vi "Write REM IO VARs.vi"(7 "R/W Case":T7, 8 "error in (no error)":errorcluster, 9 "Input FIFO buffer in":dbl[](array[numeric]), 10 "I/O Input Data In":T1 {"BD Refs"."Data Reference" format="%.0x"}, 11 "I/O Imput Vars in":T4[](array[typedef]) {"VS ref" format="%.0x"}) -> (0 "error out":errorcluster, 1 "Input FIFO buffer out":dbl[](array[numeric]), 2 "I/O Input Data Out":T1 {"BD Refs"."Data Reference" format="%.0x"}, 3 "I/O Imput Vars out":T4[](array[typedef]) {"VS ref" format="%.0x"})   [LabVIEW 2016, in "Scan Engine Custom Device.lvlib"]
uses:
  Scan Engine Custom Device.lvlib
  Type Defs/RW Case.ctl
  Type Defs/REM IO ECAT Slave IOV Cluster.ctl
  <vilib>/NI Veristand/Custom Device API/Custom Device Item Ref.ctl
  Type Defs/UDV Data Type.ctl
  Type Defs/Input Data.ctl
  <vilib>/NI Veristand/Custom Device API/Block Data Reference.ctl
  <vilib>/NI Veristand/Custom Device API/Data Reference.ctl
  <vilib>/NI Veristand/Custom Device API/Global Data Refs.vi
  <vilib>/NI Veristand/Custom Device API/Custom Device API.lvlib
  <vilib>/NI Veristand/Custom Device Tools/Custom Device Utility Library/Custom Device Utility Library.lvlib
  <vilib>/NI_Real-Time Target Support.lvlib
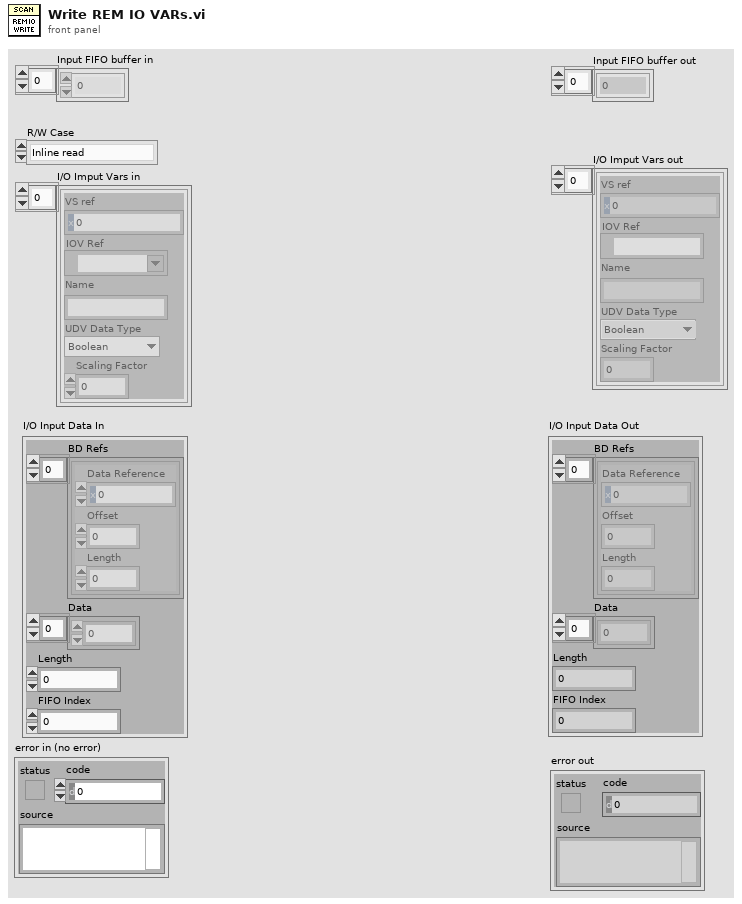
[diagram p1: front panel]
types:
  T1 = typedef "Scan Engine Custom Device.lvlib/Input Data.ctl" = cluster{"BD Refs":T2[], "Data":dbl[], "Length":i32, "FIFO Index":i32}
  T2 = typedef "Custom Device API.lvlib/Block Data Reference.ctl" = cluster{"Data Reference":T3, "Offset":u64, "Length":u64}
  T3 = typedef "Custom Device API.lvlib/Data Reference.ctl" = i32
  T4 = typedef "Scan Engine Custom Device.lvlib/REM IO ECAT Slave IOV Cluster.ctl" = cluster{"VS ref":T5, "IOV Ref":refnum<k21>, "Name":string, "UDV Data Type":T6, "Scaling Factor":dbl}
  T5 = typedef "Custom Device API.lvlib/Custom Device Item Ref.ctl" = u64
  T6 = typedef "Scan Engine Custom Device.lvlib/UDV Data Type.ctl" = enum16{"Boolean", "Fixed Point", "Int8", "Int16", "Int32", "Int64", "U32 Bit Field", "UInt8", "UInt16", "UInt32", "UInt64", "Other"}
  T7 = typedef "Scan Engine Custom Device.lvlib/RW Case.ctl" = enum16{"Inline read", "Inline write", "Async - Inline loop read", "Async - Inline loop write", "Async loop (read/write)"}
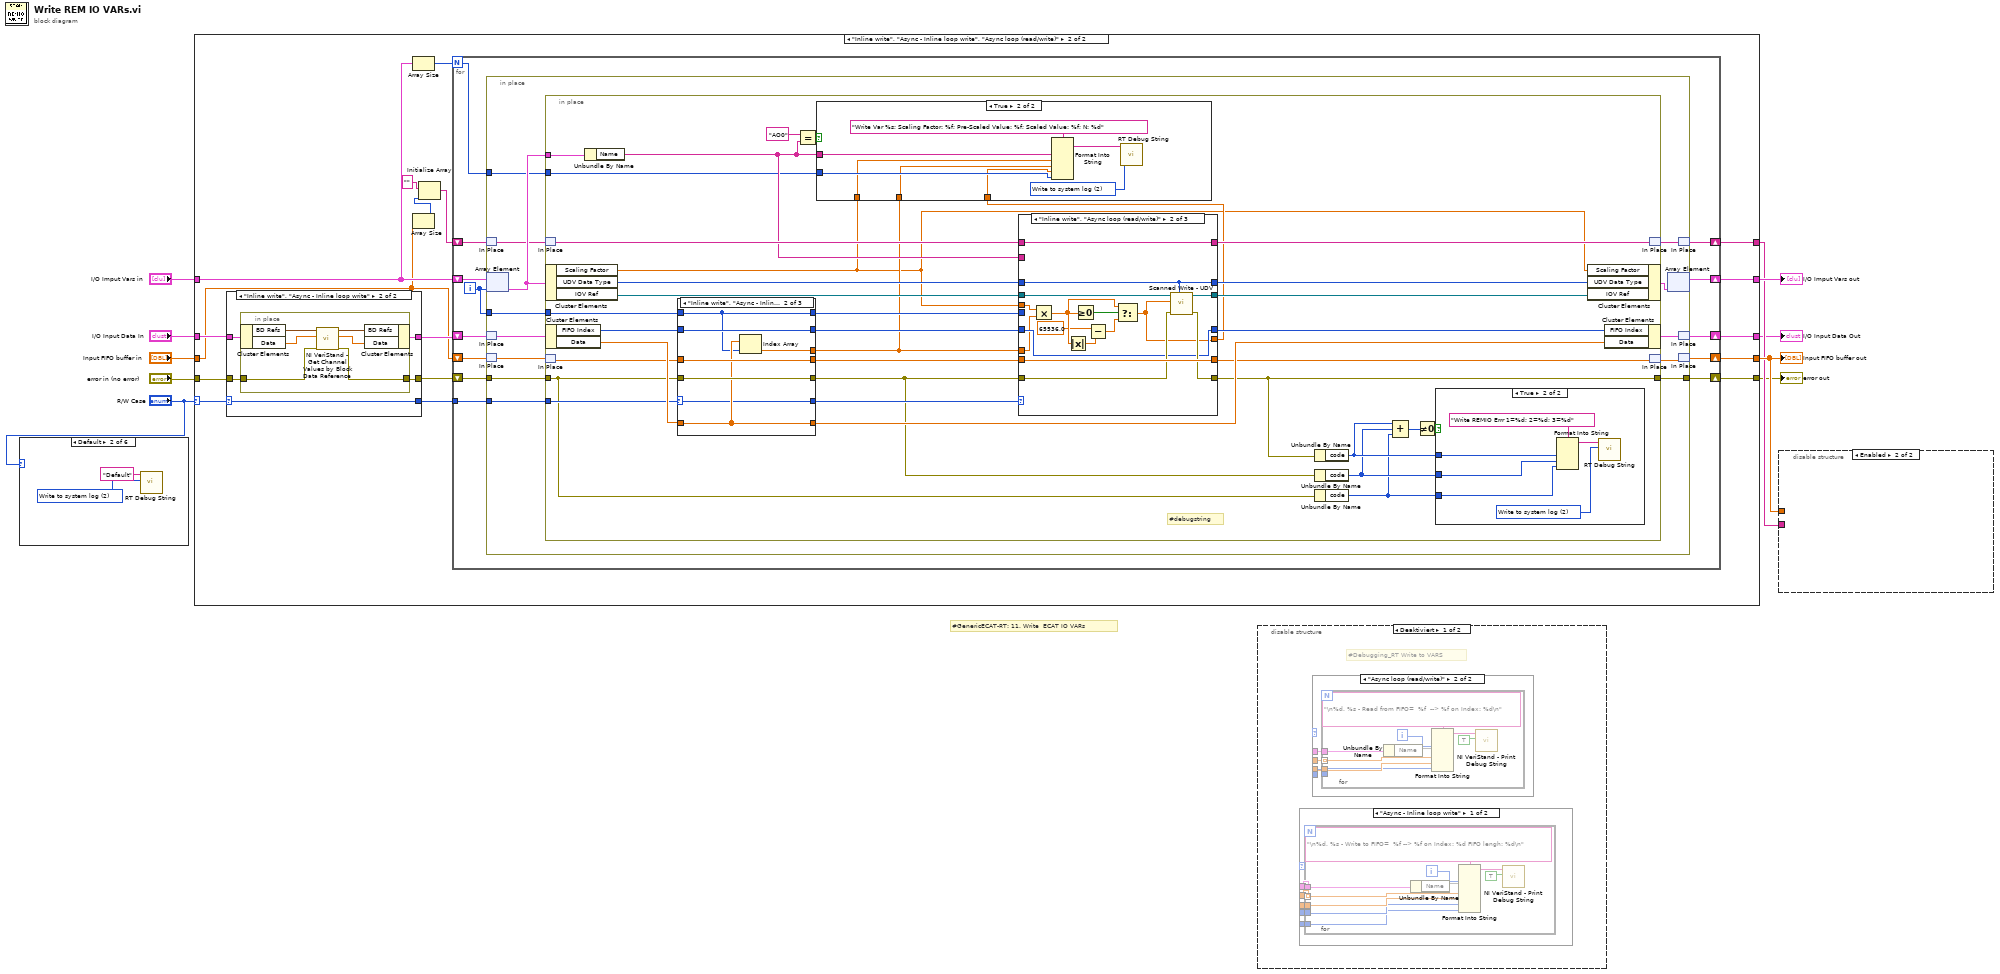
[diagram p0: block diagram]
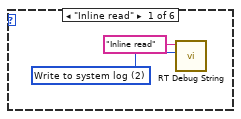
[diagram p2: hidden frame]
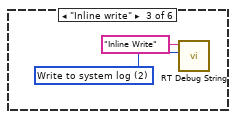
[diagram p3: hidden frame]
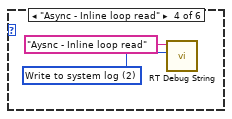
[diagram p4: hidden frame]
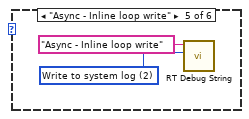
[diagram p5: hidden frame]
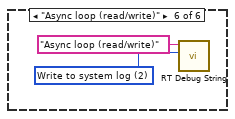
[diagram p6: hidden frame]
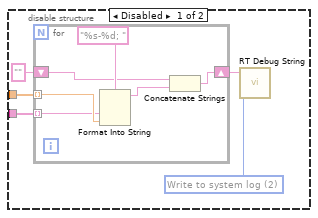
[diagram p7: hidden frame]
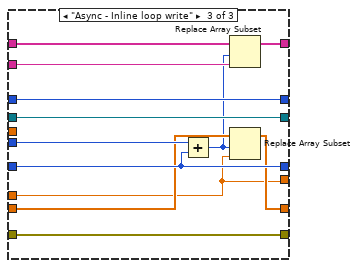
[diagram p12: hidden frame]
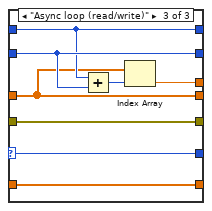
[diagram p14: hidden frame]
diagram:
  # "#GenericECAT-RT: 11. Write  ECAT IO VARs"
  n1 = case shown="Default" "R/W Case" {
    frame "Inline read" {
      w11 = u16 2 items=["Write to serial", "Write to monitor", "Write to system log"] ("Interface")
      n2 = call <vilib>:"RT Debug String.vi"("Interface"=w11, "String to write"="Inline read") -> ()  [unwired: 9 in, 1 out]
    }
    frame Default {
      w14 = u16 2 items=["Write to serial", "Write to monitor", "Write to system log"] ("Interface")
      n3 = call <vilib>:"RT Debug String.vi"("Interface"=w14, "String to write"="Default") -> ()  [unwired: 9 in, 1 out]
    }
    frame "Inline write" {
      w16 = u16 2 items=["Write to serial", "Write to monitor", "Write to system log"] ("Interface")
      n4 = call <vilib>:"RT Debug String.vi"("Interface"=w16, "String to write"="Inline Write") -> ()  [unwired: 9 in, 1 out]
    }
    frame "Async - Inline loop read" {
      w18 = u16 2 items=["Write to serial", "Write to monitor", "Write to system log"] ("Interface")
      n5 = call <vilib>:"RT Debug String.vi"("Interface"=w18, "String to write"="Aysnc - Inline loop read") -> ()  [unwired: 9 in, 1 out]
    }
    frame "Async - Inline loop write" {
      w19 = u16 2 items=["Write to serial", "Write to monitor", "Write to system log"] ("Interface")
      n6 = call <vilib>:"RT Debug String.vi"("Interface"=w19, "String to write"="Async - Inline loop write") -> ()  [unwired: 9 in, 1 out]
    }
    frame "Async loop (read/write)" {
      w21 = u16 2 items=["Write to serial", "Write to monitor", "Write to system log"] ("Interface")
      n7 = call <vilib>:"RT Debug String.vi"("Interface"=w21, "String to write"="Async loop (read/write)") -> ()  [unwired: 9 in, 1 out]
    }
  }
  n8 = case shown="\"Inline write\", \"Async - Inline loop write\", \"Async loop (read/write)\"" "R/W Case" {
    selector: "R/W Case" -> [_ w39]
    tunnel: [w24 w43] -> w6
    tunnel: "Input FIFO buffer in" -> [w24 w31]
    tunnel: [w25 w33] -> w2
    tunnel: [w26 w42] -> w7
    tunnel: "I/O Input Data In" -> [w25 w37]
    tunnel: "I/O Imput Vars in" -> [w26 w41]
    tunnel: [w23 w32] -> w4
    tunnel: "error in (no error)" -> [w23 w38]
    tunnel: [_ w28] -> w5
    frame Default {
    }
    frame "Inline write", "Async - Inline loop write", "Async loop (read/write)" {
      n9 = case shown="\"Inline write\", \"Async - Inline loop write\"" w39 {
        selector: w39 -> [w174 w177]
        tunnel: w37 -> [w175 w181]
        tunnel: w38 -> [w176 w180]
        tunnel: [w176 w179] -> w35
        tunnel: [w175 w178] -> w36
        tunnel: [w174 w177] -> w34
        frame Default {
        }
        frame "Inline write", "Async - Inline loop write" {
          n10 = in-place {
            in-place-border: w180 -> [w183]
            in-place-border: [w182] -> w179
            n11 = in-place-cluster #1(w181) -> ("BD Refs"=w187:T2[], "Data"=w185:dbl[])
            n12 = call <vilib>:"NI VeriStand - Get Channel Values by Block Data Reference.vi"("error in (no error)"=w183, "Values Array in"=w185, "Block Data Ref"=w187) -> ("error out"=w182:errorcluster, "Values Array out"=w184:dbl[], "Block Data Ref dup"=w186:T2[])  [unwired: 6 in]
            n13 = in-place-cluster #1("BD Refs"=w186, "Data"=w184) -> (w178:T1)
          }
        }
      }
      n14 = Array Size(array=w41) -> (size(s)=w40:i32)
      n15 = Array Size(array=w31) -> (size(s)=w30:i32)
      n16 = Initialize Array("", w30) -> (w27:string[])
      n17 = for {
        N: w40 -> [w44]
        shift-right: [w55] -> w42
        shift-left: w41 -> [w56]
        shift-right: [w47] -> w33
        shift-left: w36 -> [w50]
        shift-right: [w53] -> w43
        shift-left: w31 -> [w54]
        shift-right: [w51] -> w32
        shift-left: w35 -> [w52]
        tunnel: w34 -> [w49]
        shift-right: [w46] -> w28
        shift-left: w27 -> [w45]
        i -> [w48]
        n18 = in-place {
          in-place-border: w52 -> [w67]
          in-place-border: [w61] -> w51
          in-place-border: w49 -> [w66]
          in-place-border: w48 -> [w65]
          in-place-border: w44 -> [w57]
          n19 = in-place-match #2(w45) -> (w59:string[])
          n20 = in-place-array #3(w56, w48) -> (w60:T4)
          n21 = in-place-match #4(w50) -> (w69:T1)
          n22 = in-place-match #5(w54) -> (w68:dbl[])
          n23 = in-place {
            in-place-border: w67 -> [w84]
            in-place-border: w66 -> [w91]
            in-place-border: w65 -> [w102]
            in-place-border: [w82] -> w61
            in-place-border: w60 -> [w89]
            in-place-border: w57 -> [w73]
            # "#debugstring"
            n24 = in-place-match #6(w59) -> (w87:string[])
            n25 = in-place-cluster #7(w60) -> ("Scaling Factor"=w70:dbl, "UDV Data Type"=w88:T6, "IOV Ref"=w97:refnum<k21>)
            n26 = in-place-cluster #8(w69) -> ("FIFO Index"=w85:i32, "Data"=w103:dbl[])
            n27 = in-place-match #9(w68) -> (w93:dbl[])
            n28 = Unbundle By Name(w89) -> ("Name"=w76:string)
            n29 = case shown="\"Inline write\", \"Async - Inline loop write\"" w91 {
              selector: w91 -> [w155 w160 w169]
              tunnel: w102 -> [w153 w161 w170]
              tunnel: w85 -> [w158 w163 w171]
              tunnel: w93 -> [w156 w164 w168]
              tunnel: w84 -> [w154 w165 w173]
              tunnel: w103 -> [w157 w162 w172]
              tunnel: [w158 w163 w171] -> w98
              tunnel: [w157 w162 w172] -> w94
              tunnel: [w154 w165 w173] -> w83
              tunnel: [w156 w164 w168] -> w90
              tunnel: [w155 w160 w169] -> w96
              tunnel: [_ w159 w167] -> w72
              tunnel: [w153 w161 w170] -> w95
              frame Default {
              }
              frame "Inline write", "Async - Inline loop write" {
                n30 = Index Array(array=w162, index=w161) -> (element=w159:dbl)
              }
              frame "Async loop (read/write)" {
                n31 = Add(x=w170, y=w171) -> (x+y=w166:i32)
                n32 = Index Array(array=w168, index=w166) -> (element=w167:dbl)
              }
            }
            n33 = Equal?(x="AO0", y=w76) -> (x = y?=w74:bool)
            n34 = case shown="\"Inline write\", \"Async loop (read/write)\"" w96 {
              tunnel: w88 -> [w120 w137 w152]
              tunnel: w97 -> [w121 w139 w147]
              tunnel: w98 -> [w122 w128 w149]
              tunnel: w90 -> [w123 w140 w148]
              tunnel: [w123 w140 w146] -> w92
              tunnel: w95 -> [_ _ w150]
              tunnel: [w122 w128 w149] -> w99
              tunnel: [w121 w138 w147] -> w100
              tunnel: [w120 w137 w152] -> w101
              tunnel: w83 -> [w124 w136 w151]
              tunnel: [w124 w135 w151] -> w82
              tunnel: w72 -> [w118 w125 w141]
              tunnel: w87 -> [w119 w134 w145]
              tunnel: w76 -> [_ _ w143]
              tunnel: [w119 w134 w144] -> w86
              tunnel: w70 -> [_ w126 _]
              tunnel: [w118 w127 w141] -> w71
              frame Default {
              }
              frame "Inline write", "Async loop (read/write)" {
                n35 = Multiply(x=w126, y=w125) -> (x*y=w133:dbl)
                n36 = Absolute Value(x=w133) -> (abs(x)=w132:dbl)
                n37 = Greater Or Equal To 0?(x=w133) -> (x >= 0?=w129:bool)
                n38 = Subtract(x=65536.0 ("scaled data"), y=w132) -> (x-y=w131:dbl)
                n39 = Select(t=w133, s=w129, f=w131) -> (s? t:f=w127:dbl)
                n40 = call "Scanned Write - UDV.vi"("UDV Data Type"=w137, "error in (no error)"=w136, "data in"=w127, "IOV ref in"=w139) -> ("error out"=w135:errorcluster, "IOV ref out"=w138:refnum<k21>)  [unwired: 6 in]
              }
              frame "Async - Inline loop write" {
                n41 = Add(x=w150, y=w149) -> (x+y=w142:i32)
                n42 = Replace Array Subset(array=w145, new element=w143, index=w142) -> (w144:string[])
                n43 = Replace Array Subset(array=w148, new element=w141, index=w142) -> (w146:dbl[])
              }
            }
            n44 = case shown="True" w74 {
              tunnel: w72 -> [_ w104]
              tunnel: w71 -> [_ w106]
              tunnel: w76 -> [_ w111]
              tunnel: w73 -> [_ w107]
              tunnel: w70 -> [_ w105]
              frame False {
              }
              frame True {
                w110 = u16 2 items=["Write to serial", "Write to monitor", "Write to system log"] ("Interface")
                n45 = Format Into String(format string="Write Var %s; Scaling Factor: %f; Pre-Scaled Value: %f; Scaled Value: %f; N: %d", w111, w105, w104, w106, w107) -> (resulting string=w109:string)  [unwired: 2 in, 1 out]
                n46 = call <vilib>:"RT Debug String.vi"("Interface"=w110, "String to write"=w109) -> ()  [unwired: 9 in, 1 out]
              }
            }
            n47 = Unbundle By Name(w82) -> ("code"=w79:i32)
            n48 = Unbundle By Name(w83) -> ("code"=w78:i32)
            n49 = Unbundle By Name(w84) -> ("code"=w77:i32)
            n50 = Compound Arithmetic op=ADD(w79, w78, w77) -> (w81:i32)
            n51 = Not Equal To 0?(x=w81) -> (x != 0?=w80:bool)
            n52 = case shown="True" w80 {
              tunnel: w79 -> [_ w117]
              tunnel: w78 -> [_ w116]
              tunnel: w77 -> [_ w115]
              frame False {
              }
              frame True {
                w112 = u16 2 items=["Write to serial", "Write to monitor", "Write to system log"] ("Interface")
                n53 = Format Into String(format string="Write REMIO Errr 1=%d; 2=%d; 3=%d", w117, w116, w115) -> (resulting string=w113:string)  [unwired: 2 in, 1 out]
                n54 = call <vilib>:"RT Debug String.vi"("Interface"=w112, "String to write"=w113) -> ()  [unwired: 9 in, 1 out]
              }
            }
            n55 = in-place-cluster #7("Scaling Factor"=w70, "UDV Data Type"=w101, "IOV Ref"=w100) -> (w64:T4)
            n56 = in-place-cluster #8("FIFO Index"=w99, "Data"=w94) -> (w63:T1)
            n57 = in-place-match #6(w86) -> (w58:string[])
            n58 = in-place-match #9(w92) -> (w62:dbl[])
          }
          n59 = in-place-array #3(w64) -> (w55:T4[])  [unwired: 1 out]
          n60 = in-place-match #2(w58) -> (w46:string[])
          n61 = in-place-match #4(w63) -> (w47:T1)
          n62 = in-place-match #5(w62) -> (w53:dbl[])
        }
      }
    }
  }
  "Input FIFO buffer out" <- w6
  "error out" <- w4
  "I/O Imput Vars out" <- w7
  "I/O Input Data Out" <- w2
  n63 = disable-structure shown="Deaktiviert" {
    frame Disabled {
      # "#Debugging_RT Write to VARS"
      n64 = case shown="\"Async - Inline loop write\"" {
        selector: _ -> [_ _]
        tunnel: _ -> [w205 _]
        tunnel: _ -> [w204 _]
        tunnel: _ -> [w203 _]
        tunnel: _ -> [w202 _]
        tunnel: _ -> [w201 _]
        frame "Async - Inline loop write" {
          n65 = for {
            tunnel: w205 -> [w211]
            tunnel: w204 -> [w210] mode=indexing
            tunnel: w203 -> [w208]
            tunnel: w202 -> [w207]
            tunnel: w201 -> [w206]
            i -> [w213]
            n66 = Unbundle By Name(w211) -> ("Name"=w212)
            n67 = Format Into String(format string="\n%d. %s - Write to FIFO=  %f --> %f on Index: %d FIFO lengh: %d\n" ("Format-String"), w213, w212, w210, w208, w207, w206) -> (resulting string=w214:string)  [unwired: 2 in, 1 out]
            n68 = call <vilib>:"NI VeriStand - Print Debug String.vi"("Add to log file? (T)"=TRUE, "Message"=w214) -> ()  [unwired: 9 in, 1 out]
          }
        }
        frame Default {
        }
      }
      n69 = case shown="\"Async loop (read/write)\"" {
        selector: _ -> [_ _]
        tunnel: _ -> [_ w191]
        tunnel: _ -> [_ w190]
        tunnel: _ -> [_ w189]
        tunnel: _ -> [_ w188]
        frame "Async - Inline loop write", Default {
        }
        frame "Async loop (read/write)" {
          n70 = for {
            tunnel: w191 -> [w195]
            tunnel: w190 -> [w194] mode=indexing
            tunnel: w189 -> [w193]
            tunnel: w188 -> [w192]
            i -> [w197]
            n71 = Unbundle By Name(w195) -> ("Name"=w196)
            n72 = Format Into String(format string="\n%d. %s - Read from FIFO=  %f  --> %f on Index: %d\n" ("Format-String"), w197, w196, w194, w193, w192) -> (resulting string=w198:string)  [unwired: 2 in, 1 out]
            n73 = call <vilib>:"NI VeriStand - Print Debug String.vi"("Add to log file? (T)"=TRUE, "Message"=w198) -> ()  [unwired: 9 in, 1 out]
          }
        }
      }
    }
    frame Enabled {
    }
  }
  n74 = disable-structure shown="Enabled" {
    disable-tunnel: w6 -> [w220 _]
    disable-tunnel: w5 -> [w216 _]
    frame Disabled {
      w217 = u16 2 items=["Write to serial", "Write to monitor", "Write to system log"] ("Interface")
      n75 = for {
        tunnel: w220 -> [w222] mode=indexing
        shift-right: [w223] -> w218
        shift-left: "" -> [w225]
        tunnel: w216 -> [w221] mode=indexing
        n76 = Format Into String(format string="%s-%d; ", w221, w222) -> (resulting string=w224:string)  [unwired: 2 in, 1 out]
        n77 = Concatenate Strings(w225, w224) -> (w223:string)
      }
      n78 = call <vilib>:"RT Debug String.vi"("Interface"=w217, "String to write"=w218) -> ()  [unwired: 9 in, 1 out]
    }
    frame Enabled {
    }
  }
